vi "Waveform Chart.vi"() -> ()   [LabVIEW 2020]
panel:
  in  "Stop":bool
  in  "UpdateTime(ms)":i32=200
  out "Waveform Chart - Light":T1(graph)={"number: 0 to 1"=0.6519846813155175, "number: 0 to 1"=0.8352194486753195, "number: 0 to 1"=0.06686301033922293, "number: 0 to 1"=0.9204713202449457, "number: 0 to 1"=0.5179307849850288, "number: 0 to 1"=0.1224884132279076, "number: 0 to 1"=0.15735162584891316, "number: 0 to 1"=0.2750388048209973}
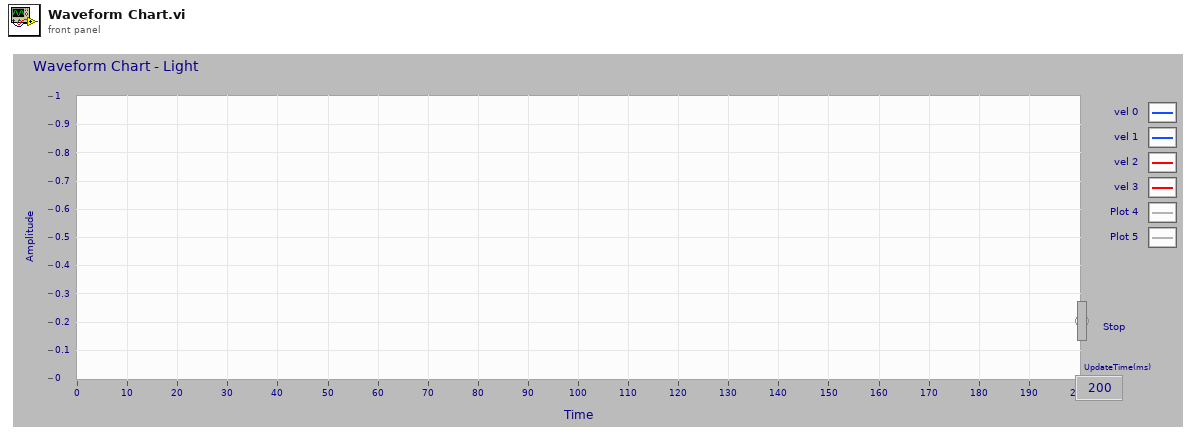
[diagram p1: front panel]
types:
  T1 = cluster{"number: 0 to 1":dbl, "number: 0 to 1":dbl, "number: 0 to 1":dbl, "number: 0 to 1":dbl, "number: 0 to 1":dbl, "number: 0 to 1":dbl, "number: 0 to 1":dbl, "number: 0 to 1":dbl}
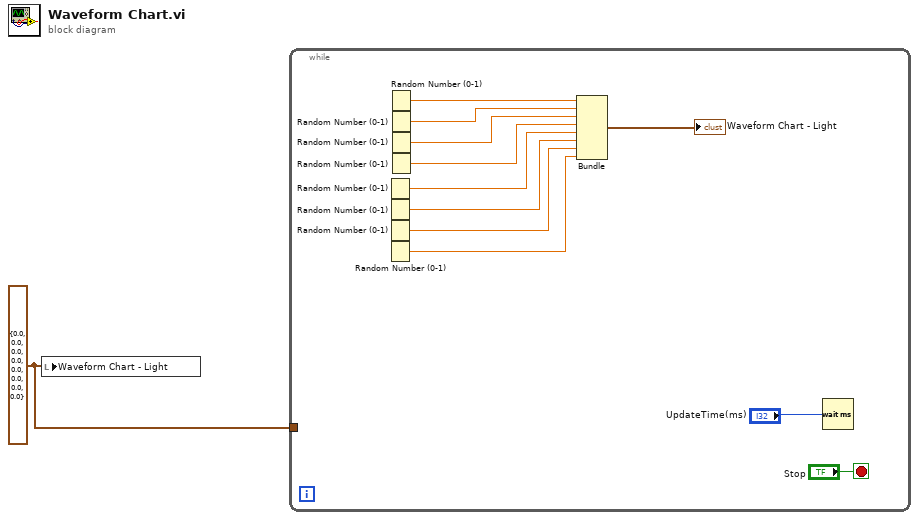
[diagram p0: block diagram]
diagram:
  w1 = T1 {"number: 0 to 1"=0.0, "number: 0 to 1"=0.0, "number: 0 to 1"=0.0, "number: 0 to 1"=0.0, "number: 0 to 1"=0.0, "number: 0 to 1"=0.0, "number: 0 to 1"=0.0, "number: 0 to 1"=0.0} ("Waveform Chart - Light")
  n1 = local write "Waveform Chart - Light"(w1) -> ()
  n2 = while {
    tunnel: w1 -> [_]
    stop <- "Stop" stop-if-true
    n3 = Random Number (0-1)() -> (number: 0 to 1=w7:dbl)
    n4 = Random Number (0-1)() -> (number: 0 to 1=w6:dbl)
    n5 = Random Number (0-1)() -> (number: 0 to 1=w5:dbl)
    n6 = Random Number (0-1)() -> (number: 0 to 1=w4:dbl)
    n7 = Random Number (0-1)() -> (number: 0 to 1=w12:dbl)
    n8 = Random Number (0-1)() -> (number: 0 to 1=w11:dbl)
    n9 = Random Number (0-1)() -> (number: 0 to 1=w10:dbl)
    n10 = Random Number (0-1)() -> (number: 0 to 1=w9:dbl)
    n11 = Bundle("number: 0 to 1"=w12, "number: 0 to 1"=w11, "number: 0 to 1"=w10, "number: 0 to 1"=w9, "number: 0 to 1"=w7, "number: 0 to 1"=w6, "number: 0 to 1"=w5, "number: 0 to 1"=w4) -> (→"Waveform Chart - Light":T1)  [unwired: 1 in]
    n12 = Wait (ms)(milliseconds to wait="UpdateTime(ms)") -> ()  [unwired: 1 out]
  }
